vi "tcsWEP_acceptCommand_disable.vi"(8 "error in (no error)":errorcluster, 11 "command_disable_Ctl":T1) -> (0 "error out":errorcluster, 2 "function return":i32, 3 "command_disable_Ctl out":T1)   [LabVIEW 2016, in "SALLV_tcsWEP.lvlib"]
doc: "int tcsWEP_shm_acceptCommand_disableLV(tcsWEP_command_disableLV *command_disable_Ctl );"
uses:
  SALLV_tcsWEP.lvlib
  DataTypes/command_disable.ctl
  SALLV_tcsWEP.so
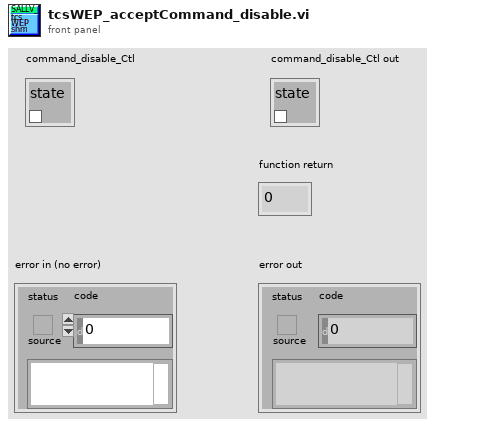
[diagram p1: front panel]
types:
  T1 = typedef "SALLV_tcsWEP.lvlib/command_disable.ctl" = cluster{"state":bool}
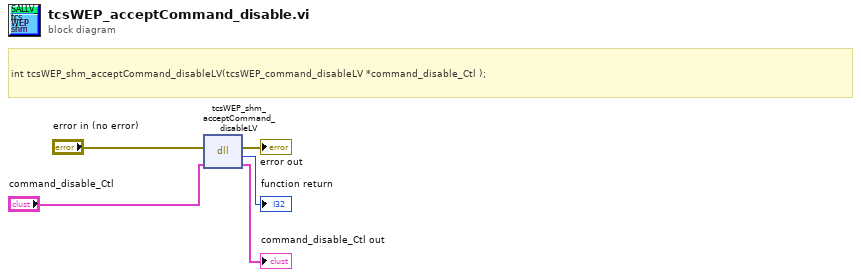
[diagram p0: block diagram]
diagram:
  # "int tcsWEP_shm_acceptCommand_disableLV(tcsWEP_command_disableLV *command_disable_Ctl );"
  n1 = dll-call lib="home/ttsai/Documents/salAPI/SALLV_tcsWEP.*" fn="tcsWEP_shm_acceptCommand_disableLV"(error in="error in (no error)", "command_disable_Ctl"="command_disable_Ctl") -> (error out=→"error out":errorcluster, →"function return":i32, "command_disable_Ctl"=→"command_disable_Ctl out":T1)  [unwired: 2 in, 1 out]
